vi "Wrapper_setIntegrationTime.vi"(1 "Integration Time":i32, 2 "Index":i32, 3 "Wrapper In":u32) -> (0 "Wrapper Out":u32)   [LabVIEW 2012]
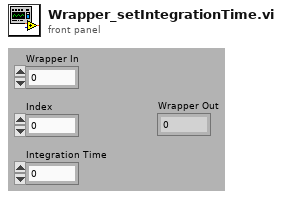
[diagram p1: front panel]
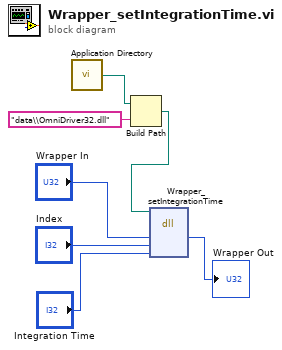
[diagram p0: block diagram]
diagram:
  n1 = call <vilib>:"Application Directory.vi"() -> ("Application Directory"=w3:path)
  n2 = Build Path(base path=w3, name or relative path="data\\OmniDriver32.dll") -> (appended path=w1:path)
  n3 = dll-call lib="D:/Software Development/EPI Development/BurnIn Testing/Instruments/Drivers/Ocean Optics/OOI_HOME/OmniDriver32.dll" fn="Wrapper_setIntegrationTime" label="Wrapper.setIntegrationTime"(path in=w1, "Wrapper"="Wrapper In", "Index"="Index", "Integration Time"="Integration Time") -> ("Wrapper"=→"Wrapper Out":u32)  [unwired: 4 in, 3 out]
